vi "Match-Value Image (Colour).vi"(8 "error in (no error)":errorcluster, 9 "Value":u32(colorbox), 10 "Match in":T1, 11 "ARGB Image Source in":T2) -> (0 "error out":errorcluster, 3 "Match Destination":T1)   [LabVIEW 2020, in "image.lvlib"]
doc: "Compute a single channel image which will contain non-zero pixels for any pixel in the Source Image which matches the given value.\n\nThis is similar to Image \"In-Range\" but only matches a single value."
uses:
  image.lvlib
  ARGB Image.ctl
  Greyscale Image.ctl
  5701baee-35e2-4306-9a77-a9fdbb5b3a7f.vi
  <vilib>/Utility/error.llb/Error Cluster From Error Code.vi
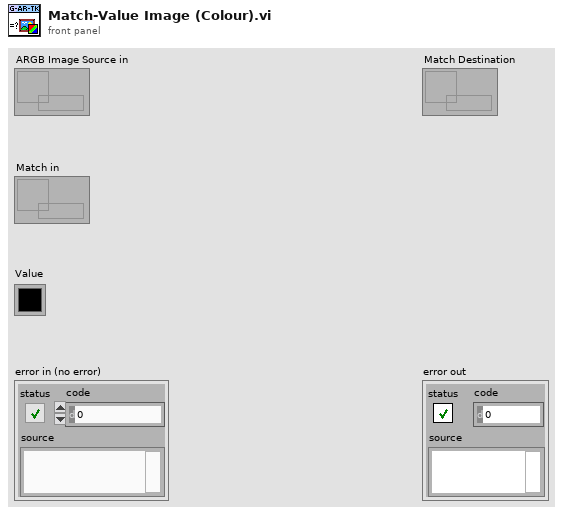
[diagram p1: front panel]
types:
  T1 = typedef "image.lvlib/Greyscale Image.ctl" = refnum<data-value>
  T2 = typedef "image.lvlib/ARGB Image.ctl" = refnum<data-value>
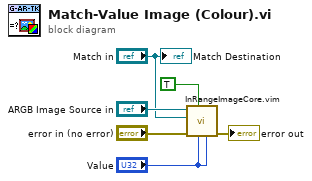
[diagram p0: block diagram]
diagram:
  n1 = call "InRangeImageCore.vim"("Upper"="Value", "Lower"="Value", "IgnoreAlpha"=TRUE, "error in (no error)"="error in (no error)", "In-Range-Result"="Match in", "Src"="ARGB Image Source in") -> ("error out"=→"error out":errorcluster)  [unwired: 5 in]
  "Match Destination" <- "Match in"
